vi "Test mysql queries.vi"() -> ()   [LabVIEW 2020, in "mysql-queries.lvlib" / "mysql-queries.lvclass"]
uses:
  mysql-queries.lvclass
  externals/mysql/Source/mysql.net/mysql.lvclass
panel:
  out "Result":string
  out "error out":errorcluster
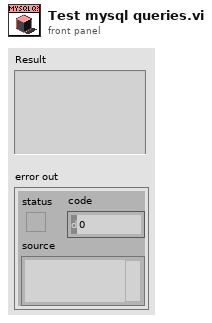
[diagram p1: front panel]
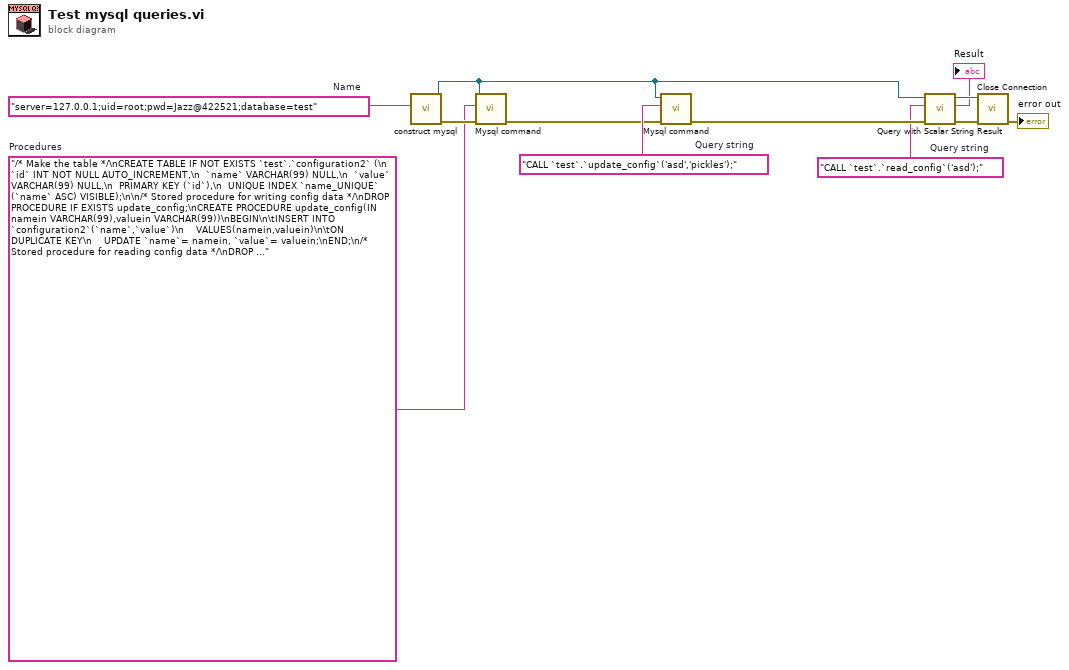
[diagram p0: block diagram]
diagram:
  w9 = "CALL `test`.`read_config`('asd');"  # Query string
  w11 = "CALL `test`.`update_config`('asd','pickles');"  # Query string
  w2 = "/* Make the table */\nCREATE TABLE IF NOT EXISTS `test`.`configuration2` (\n  `id` INT NOT NULL AUTO_INCREMENT,\n  `name` VARCHAR(99) NULL,\n  `value` VARCHAR(99) NULL,\n  PRIMARY KEY (`id`),\n  UNIQUE INDEX `name_UNIQUE` (`name` ASC) VISIBLE);\n\n/* Stored procedure for writing config data */\nDROP PROCEDURE IF EXISTS update_config;\nCREATE PROCEDURE update_config(IN namein VARCHAR(99),valuein VARCHAR(99))\nBEGIN\n\tINSERT INTO `configuration2`(`name`,`value`)\n    VALUES(namein,valuein)\n\tON DUPLICATE KEY\n    UPDATE `name`= namein, `value`= valuein;\nEND;\n/* Stored procedure for reading config data */\nDROP procedure IF EXISTS `read_config`;\nCREATE PROCEDURE read_config(IN namein VARCHAR(99))\nBEGIN\n\tSELECT `value` FROM `configuration`.`configuration2` WHERE `name`=namein;\nEND;"  # Procedures
  w12 = "server=127.0.0.1;uid=root;pwd=Jazz@422521;database=test"  # Name
  n1 = call "construct mysql.vi"("Connection string"=w12) -> ("error out"=w4:errorcluster, "mysql out"=w1:refnum<class "mysql.lvclass">)  [unwired: 9 in]
  n2 = call "Mysql command.vi"("error in (no error)"=w4, "Query string"=w2, "mysql in"=w1) -> ("error out"=w3:errorcluster)  [unwired: 7 in, 1 out]
  n3 = call "Mysql command.vi"("error in (no error)"=w3, "Query string"=w11, "mysql in"=w1) -> ("error out"=w10:errorcluster)  [unwired: 7 in, 1 out]
  n4 = call-dynamic "Query with Scalar String Result.vi"("error in (no error)"=w10, "Query string"=w9, "mysql in"=w1) -> ("error out"=w7:errorcluster, "Result"=→"Result":string, "mysql out"=w8:refnum<class "mysql.lvclass">)  [unwired: 6 in]
  n5 = call-dynamic "Close Connection.vi"("error in (no error)"=w7, "mysql in"=w8) -> ("error out"=→"error out":errorcluster)  [unwired: 8 in, 1 out]
